vi "Conditional Terminal.vi"() -> ()   [LabVIEW 2020]
uses:
  <vilib>/Utility/sysdir.llb/System Directory Type.ctl
panel:
  in  "stop":bool
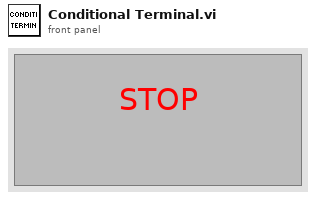
[diagram p1: front panel]
types:
  T1 = typedef "System Directory Type.ctl" = i32
  T2 = enum16{"open", "replace", "create", "open or create", "replace or create", "replace or create with confirmation"}
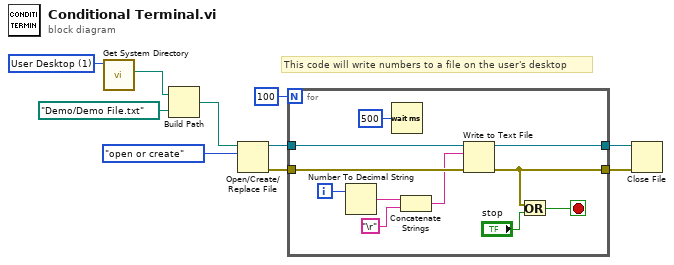
[diagram p0: block diagram]
diagram:
  w9 = T1 1 items=["User Home"=0, "User Desktop"=1, "User Documents"=2, "User Application Data"=3, "User Preferences"=4, "User Temporary"=5, "Public Documents"=6, "Public Application Data"=7, "Public Preferences"=8, "Public Cache"=13, "System Core Libraries"=9, "System Installed Libraries"=10, "Application Files"=11, "Boot Volume Root"=12] ("system directory type")
  # "This code will write numbers to a file on the user's desktop"
  n1 = call <vilib>:"Get System Directory.vi"("system directory type"=w9) -> ("system directory"=w8:path)  [unwired: 10 in]
  n2 = Build Path(base path=w8, name or relative path=path "Demo/Demo File.txt") -> (appended path=w6:path)
  n3 = Open/Create/Replace File(file path (use dialog)=w6, operation (0:open)=T2."open or create") -> (refnum out=w5:refnum<file>, error out=w4:errorcluster)  [unwired: 4 in, 1 out]
  n4 = for {
    N: 100 -> [_]
    tunnel: w5 -> [w21]
    tunnel: w4 -> [w20]
    tunnel: [w12] -> w3
    tunnel: [w19] -> w2
    i -> [w18]
    stop <- w11 stop-if-true
    n5 = Number To Decimal String(number=w18) -> (decimal integer string=w17:string)  [unwired: 1 in]
    n6 = Wait (ms)(milliseconds to wait=u32 500) -> ()  [unwired: 1 out]
    n7 = Concatenate Strings(w17, "\r") -> (w15:string)
    n8 = Write to Text File(file (use dialog)=w21, text=w15, error in=w20) -> (refnum out=w19:refnum<file>, error out=w12:errorcluster)  [unwired: 1 in, 1 out]
    n9 = Or(x=w12, y="stop") -> (x .or. y?=w11:bool)
  }
  n10 = Close File(refnum=w2, error in=w3) -> ()  [unwired: 2 out]
